vi "FPGA_Main.vi"() -> ()   [LabVIEW 2019]
uses:
  <vilib>/rvi/Emulation/niFpgaGetClockAttributes.vi
  <vilib>/rvi/Emulation/niFpgaSctlEmulationGetInTimedLoop.vi
  <vilib>/rvi/Emulation/niFpgaEmulationReportErrorSimple.vi
  <vilib>/rvi/Emulation/niFpgaCriticalErrorInLSC.vi
  <vilib>/rvi/eio/common/nirviEmuTemplateMethod_errors.vi
  <vilib>/eio/EIONode/EIONode.xnode
panel:
  out "R SPRING TORQUE":fxp<+/-,64,24>
  out "RIGHT MOTOR POS":fxp<+,51,11>
  out "RIGHT ACT POS":fxp<+,51,11>
  in  "SPRING CONST":fxp<+/-,53,13>=11.0 format="%#_44g"
  in  "ENC INIT":bool=TRUE
  out "L_CURRENT_DES":fxp<+/-,64,49>
  out "FUTEK":i16
  in  "ASSIST":bool=TRUE
  in  "L_TRQ_DES":fxp<+/-,32,16>
  in  "R_TRQ_DES":fxp<+/-,32,16>
  out "LOOP RATE":u32 caption="Tick Count(uSec)"
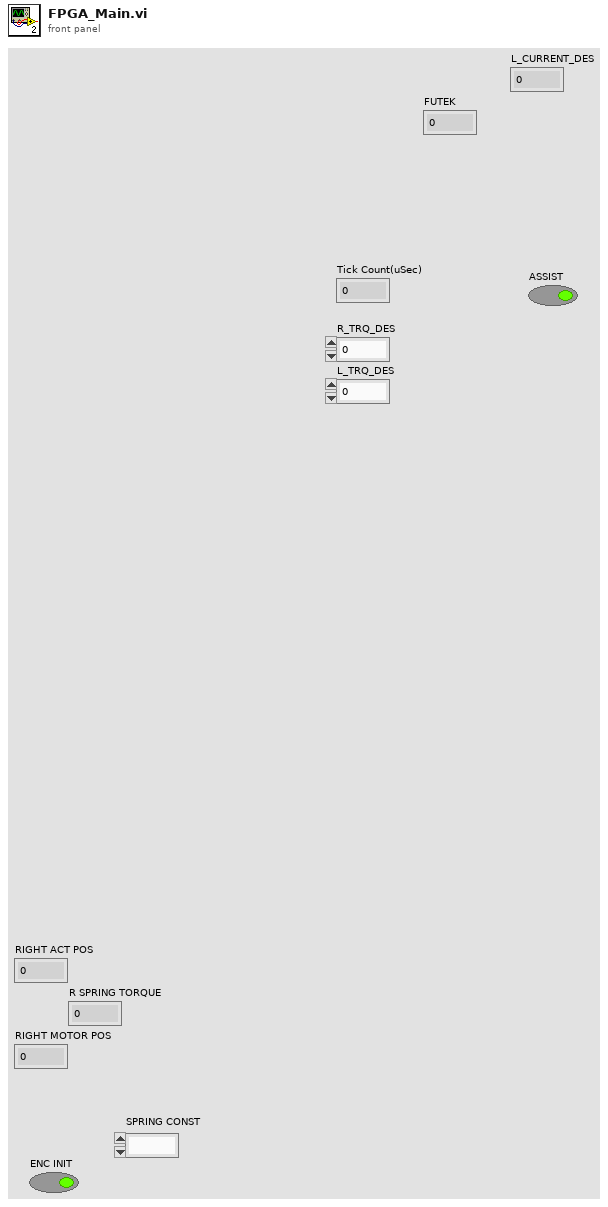
[diagram p1: front panel]
types:
  T1 = enum16{"100kBPS", "250kBPS", "500kBPS", "1000kBPS"}
  T2 = typedef "SPI Config.ctl" = cluster{"MXP Port":enum16{"A", "B"}, "Device":enum16{"CAN", "ENC", "IMU1", "IMU2"}, "CPOL":bool}
  T3 = enum32{"Duty", "Current", "Brake", "RPM", "Position"}
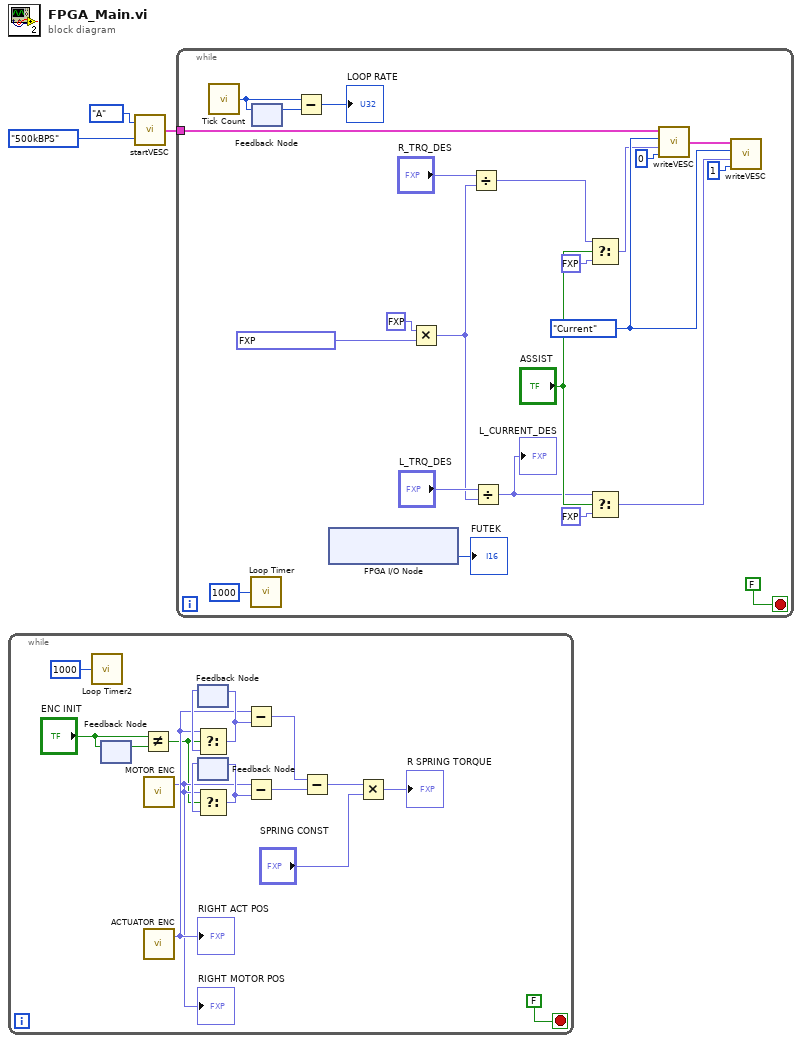
[diagram p0: block diagram]
diagram:
  n1 = while {
    stop <- FALSE stop-if-true
    n2 = call "Loop Timer2"("Count(uSec)"=u32 1000) -> ()  [unwired: 1 out]
    n3 = feedback #1() -> (w17:bool)  [unwired: 1 in]
    n4 = feedback-in #1("ENC INIT") -> ()
    n5 = Not Equal?(x="ENC INIT", y=w17) -> (x != y?=w6:bool)
    n6 = call "MOTOR ENC.vi"() -> ("RIGHT MOTOR POS"=w7:fxp<+,51,11>)  [unwired: 1 in, 1 out]
    "RIGHT MOTOR POS" <- w7
    n7 = call "ACTUATOR ENC.vi"() -> ("RIGHT ACT POS"=w8:fxp<+,51,11>)  [unwired: 1 in, 1 out]
    "RIGHT ACT POS" <- w8
    n8 = feedback #2() -> (w15:fxp<+,51,11>)  [unwired: 1 in]
    n9 = Select(t=w8, s=w6, f=w15) -> (s? t:f=w14:fxp<+,51,11>)
    n10 = feedback-in #2(w14) -> ()
    n11 = feedback #3() -> (w13:fxp<+,51,11>)  [unwired: 1 in]
    n12 = Select(t=w7, s=w6, f=w13) -> (s? t:f=w12:fxp<+,51,11>)
    n13 = feedback-in #3(w12) -> ()
    n14 = Subtract(x=w8, y=w14) -> (x-y=w10:fxp<+/-,52,12>)
    n15 = Subtract(x=w7, y=w12) -> (x-y=w11:fxp<+/-,52,12>)
    n16 = Subtract(x=w10, y=w11) -> (x-y=w9:fxp<+/-,53,13>)
    n17 = Multiply(x=w9, y="SPRING CONST") -> (x*y=→"R SPRING TORQUE":fxp<+/-,64,25>)
  }
  n18 = call "startVESC.vi"("Baud Rate"=T1."500kBPS", "MXP Port"=enum16{"A", "B"}."A") -> ("SPI Config Out"=w3:T2)
  n19 = while {
    tunnel: w3 -> [w37]
    stop <- FALSE stop-if-true
    w33 = T3."Current" ("Control Mode")
    n20 = call "Tick Count"() -> ("Tick Count(uSec)"=w40:u32)
    n21 = call "Loop Timer"("Count(uSec)"=u32 1000) -> ()  [unwired: 1 out]
    n22 = feedback-in #4(w40) -> ()
    n23 = feedback #4() -> (w39:u32)  [unwired: 1 in]
    n24 = Subtract(x=w40, y=w39) -> (x-y=→"LOOP RATE":u32)
    n25 = xnode "FPGA I/O Node"() -> ("ConnectorC/AI1"=→"FUTEK":i16)  [unwired: 1 in, 1 out]
    n26 = Multiply(x=fxp<+/-,32,16> 50.0 ("f"), y=fxp<+/-,32,16> 0.09100341796875) -> (x*y=w22:fxp<+/-,64,32>)
    n27 = Divide(x="R_TRQ_DES", y=w22) -> (x/y=w20:fxp<+/-,64,49>)
    n28 = Divide(x="L_TRQ_DES", y=w22) -> (x/y=w21:fxp<+/-,64,49>)
    "L_CURRENT_DES" <- w21
    n29 = Select(t=w20, s="ASSIST", f=fxp<+/-,32,16> 0.0) -> (s? t:f=w32:fxp<+/-,64,49>)
    n30 = Select(t=w21, s="ASSIST", f=fxp<+/-,32,16> 0.0) -> (s? t:f=w28:fxp<+/-,64,49>)
    n31 = call "writeVESC.vi"("ID"=u32 0, "Control Value"=w32, "Control Mode"=w33, "SPI Config In"=w37) -> ("SPI Config Out"=w36:T2)
    n32 = call "writeVESC.vi"("ID"=u32 1, "Control Value"=w28, "Control Mode"=w33, "SPI Config In"=w36) -> ()  [unwired: 1 out]
  }
